vi "GenerateDataset.vi"(8 "error in (no error)":errorcluster) -> (0 "error out":errorcluster, 3 "DataSets_All(In1D_Out1D)":T1)   [LabVIEW 2020]
uses:
  <vilib>/Ngene/DeepLTK/Toolkit/NN_Data/API/DataSet_Types/NN_DataSets_All(In1D_Out1D).ctl
  <vilib>/Ngene/DeepLTK/Toolkit/NN_Data/API/DataSet_Types/NN_DataSet(In1D_Out1D).ctl
  <vilib>/Ngene/DeepLTK/Toolkit/NN_Data/API/DataRef_Types/NN_Data_ref(2D_SGL).ctl
  <vilib>/Ngene/DeepLTK/Toolkit/NN_Data/API/DataRef_Types/NN_Data_ref(1D_I32).ctl
  <vilib>/Ngene/DeepLTK/Toolkit/Deep_Learning_Toolkit_by_Ngene.lvlib
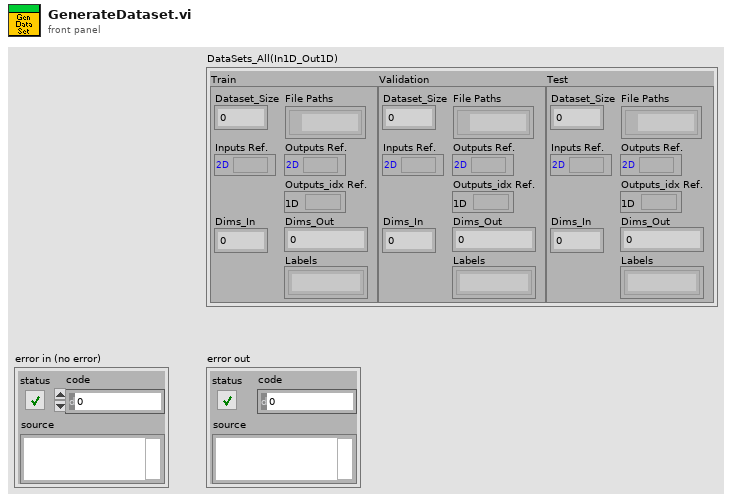
[diagram p1: front panel]
types:
  T1 = typedef "Deep_Learning_Toolkit_by_Ngene.lvlib/NN_DataSets_All(In1D_Out1D).ctl" = cluster{"Train":T2, "Validation":T2, "Test":T2}
  T2 = typedef "Deep_Learning_Toolkit_by_Ngene.lvlib/NN_DataSet(In1D_Out1D).ctl" = cluster{"Inputs Ref.":T3, "Outputs Ref.":T3, "Dims_In":i32, "Dataset_Size":i32, "Outputs_idx Ref.":T4, "Dims_Out":i32, "Labels":string[], "File Paths":path[]}
  T3 = typedef "Deep_Learning_Toolkit_by_Ngene.lvlib/NN_Data_ref(2D_SGL).ctl" = refnum<data-value>
  T4 = typedef "Deep_Learning_Toolkit_by_Ngene.lvlib/NN_Data_ref(1D_I32).ctl" = refnum<data-value>
  T5 = enum16{"Sine Wave", "Triangle Wave", "Square Wave", "Sawtooth Wave", "Noise"}[]
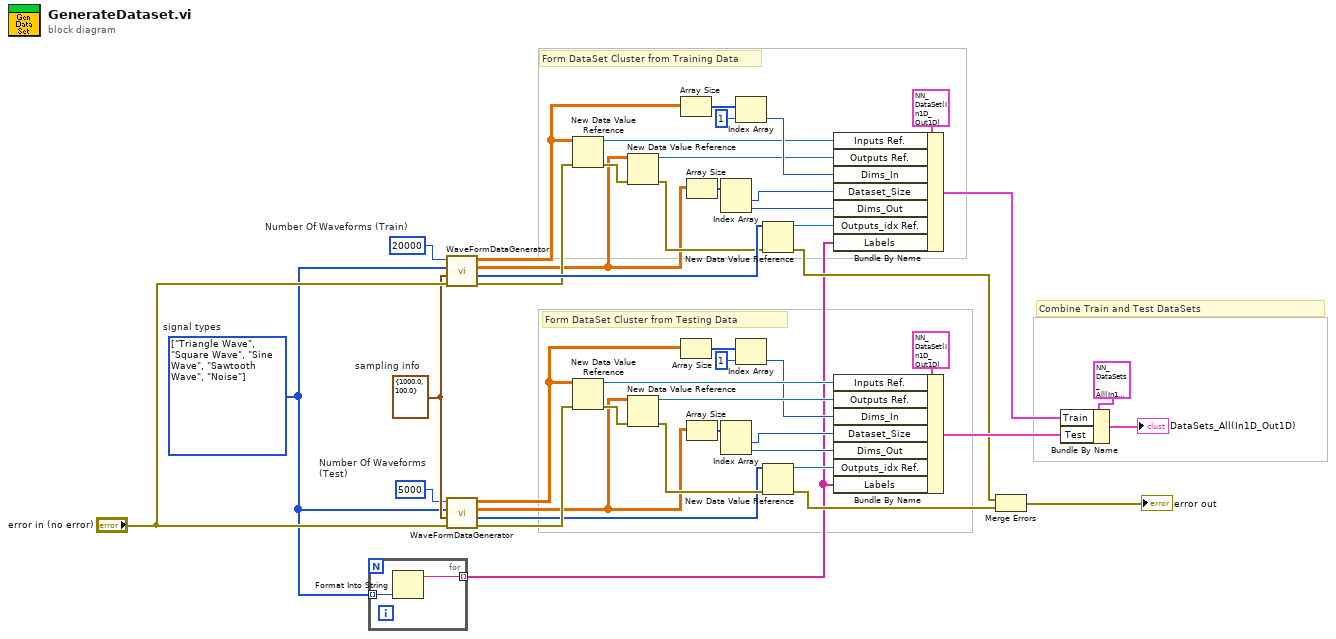
[diagram p0: block diagram]
diagram:
  w36 = 5000  # Number Of Waveforms (Test)
  w43 = cluster{"Fs":dbl, "#s":dbl} {"Fs"=1000.0, "#s"=100.0}  # sampling info
  w10 = 20000  # Number Of Waveforms (Train)
  w3 = T5 [enum."Triangle Wave", enum."Square Wave", enum."Sine Wave", enum."Sawtooth Wave", enum."Noise"] items=["Sine Wave", "Triangle Wave", "Square Wave", "Sawtooth Wave", "Noise"]  # signal types
  # "Combine Train and Test DataSets"
  # "Form DataSet Cluster from Testing Data"
  # "Form DataSet Cluster from Training Data"
  n1 = for {
    tunnel: w3 -> [w47] mode=indexing
    tunnel: [w46] -> w2 mode=indexing
    n2 = Format Into String(w47) -> (resulting string=w46:string)  [unwired: 3 in, 1 out]
  }
  n3 = call "WaveFormDataGenerator.vi"("error in"="error in (no error)", "sampling info"=w43, "Signal Types"=w3, "Number of Waveforms Per Class"=w10) -> ("error out"=w9:errorcluster, "Class Idx"=w21:i32[], "One-Hot Encoded Output"=w1:sgl[][], "Generated Waveform"=w14:sgl[][])  [unwired: 4 in]
  n4 = call "WaveFormDataGenerator.vi"("error in"="error in (no error)", "sampling info"=w43, "Signal Types"=w3, "Number of Waveforms Per Class"=w36) -> ("error out"=w37:errorcluster, "Class Idx"=w24:i32[], "One-Hot Encoded Output"=w29:sgl[][], "Generated Waveform"=w32:sgl[][])  [unwired: 4 in]
  n5 = New Data Value Reference(data value=w14, error in=w9) -> (data value reference=w13:refnum<data-value>, error out=w4:errorcluster)
  n6 = New Data Value Reference(data value=w32, error in=w37) -> (data value reference=w33:refnum<data-value>, error out=w40:errorcluster)
  n7 = New Data Value Reference(data value=w1, error in=w4) -> (data value reference=w12:refnum<data-value>, error out=w8:errorcluster)
  n8 = New Data Value Reference(data value=w29, error in=w40) -> (data value reference=w34:refnum<data-value>, error out=w38:errorcluster)
  n9 = Array Size(array=w14) -> (size(s)=w15:i32[])
  n10 = Array Size(array=w32) -> (size(s)=w31:i32[])
  n11 = Array Size(array=w1) -> (size(s)=w16:i32[])
  n12 = Array Size(array=w29) -> (size(s)=w30:i32[])
  n13 = Index Array(array=w16) -> (element #1=w20:i32, element #2=w17:i32)  [unwired: 2 in]
  n14 = Index Array(array=w30) -> (element #1=w25:i32, element #2=w28:i32)  [unwired: 2 in]
  n15 = Index Array(array=w15, index=1) -> (element=w19:i32)
  n16 = Index Array(array=w31, index=1) -> (element=w26:i32)
  n17 = New Data Value Reference(data value=w21, error in=w8) -> (data value reference=w11:refnum<data-value>, error out=w23:errorcluster)
  n18 = New Data Value Reference(data value=w24, error in=w38) -> (data value reference=w35:refnum<data-value>, error out=w41:errorcluster)
  n19 = Bundle By Name(cluster=T2 {"Inputs Ref."=refnum, "Outputs Ref."=refnum, "Dims_In"=0, "Dataset_Size"=0, "Outputs_idx Ref."=refnum, "Dims_Out"=0, "Labels"=[], "File Paths"=[]} ("Dataset(In1D_Out1D)"), "Inputs Ref."=w13, "Outputs Ref."=w12, "Dims_In"=w19, "Dataset_Size"=w20, "Dims_Out"=w17, "Outputs_idx Ref."=w11, "Labels"=w2) -> (w7:T2)
  n20 = Bundle By Name(cluster=T2 {"Inputs Ref."=refnum, "Outputs Ref."=refnum, "Dims_In"=0, "Dataset_Size"=0, "Outputs_idx Ref."=refnum, "Dims_Out"=0, "Labels"=[], "File Paths"=[]} ("Dataset(In1D_Out1D)"), "Inputs Ref."=w33, "Outputs Ref."=w34, "Dims_In"=w26, "Dataset_Size"=w25, "Dims_Out"=w28, "Outputs_idx Ref."=w35, "Labels"=w2) -> (w42:T2)
  n21 = Merge Errors(w23, w41) -> (→"error out":errorcluster)
  n22 = Bundle By Name(cluster=T1 {"Train"={"Inputs Ref."=refnum, "Outputs Ref."=refnum, "Dims_In"=0, "Dataset_Size"=0, "Outputs_idx Ref."=refnum, "Dims_Out"=0, "Labels"=[], "File Paths"=[]}, "Validation"={"Inputs Ref."=refnum, "Outputs Ref."=refnum, "Dims_In"=0, "Dataset_Size"=0, "Outputs_idx Ref."=refnum, "Dims_Out"=0, "Labels"=[], "File Paths"=[]}, "Test"={"Inputs Ref."=refnum, "Outputs Ref."=refnum, "Dims_In"=0, "Dataset_Size"=0, "Outputs_idx Ref."=refnum, "Dims_Out"=0, "Labels"=[], "File Paths"=[]}} ("DataSets_All(In1D_Out1D)"), "Train"=w7, "Test"=w42) -> (→"DataSets_All(In1D_Out1D)":T1)
